vi "Get Tuner Gain.vi"(8 "error in (no error)":errorcluster, 11 "RTL-SDR in":refnum<class "Session.lvclass">) -> (0 "error out":errorcluster, 2 "Tuner Gain":dbl, 3 "RTL-SDR out":refnum<class "Session.lvclass">)   [LabVIEW 2020, in "RTL-SDR.lvlib" / "Session.lvclass"]
uses:
  Session.lvclass
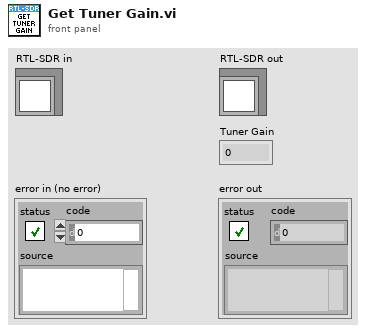
[diagram p1: front panel]
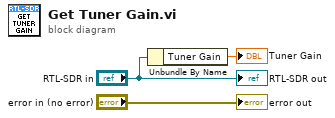
[diagram p0: block diagram]
diagram:
  n1 = Unbundle By Name("RTL-SDR in") -> ("Tuner Gain"=→"Tuner Gain":dbl)
  "error out" <- "error in (no error)"
  "RTL-SDR out" <- "RTL-SDR in"
